vi "Izhikevich_primitive_v001.vi"(0 "UDP Network Connection in":refnum<k16>, 1 "b":dbl, 2 "a":dbl, 3 "I":dbl, 5 "c":dbl, 7 "d":dbl, 9 "v(t)":dbl, 10 "Neuron ID":dbl=1.0, 11 "error in (no error)":errorcluster, 12 "u(t)":dbl, 13 "dt":dbl) -> (4 "UDP Network Connection out":refnum<k16>, 6 "v(t+dt)":dbl, 8 "u(t+dt)":dbl, 15 "error out":errorcluster)   [LabVIEW 2019]
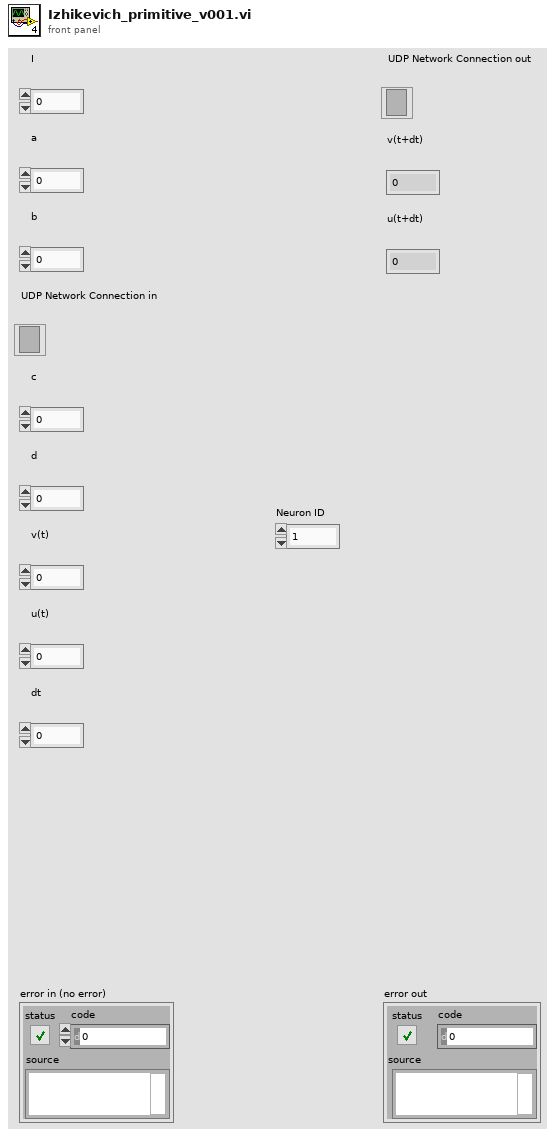
[diagram p1: front panel]
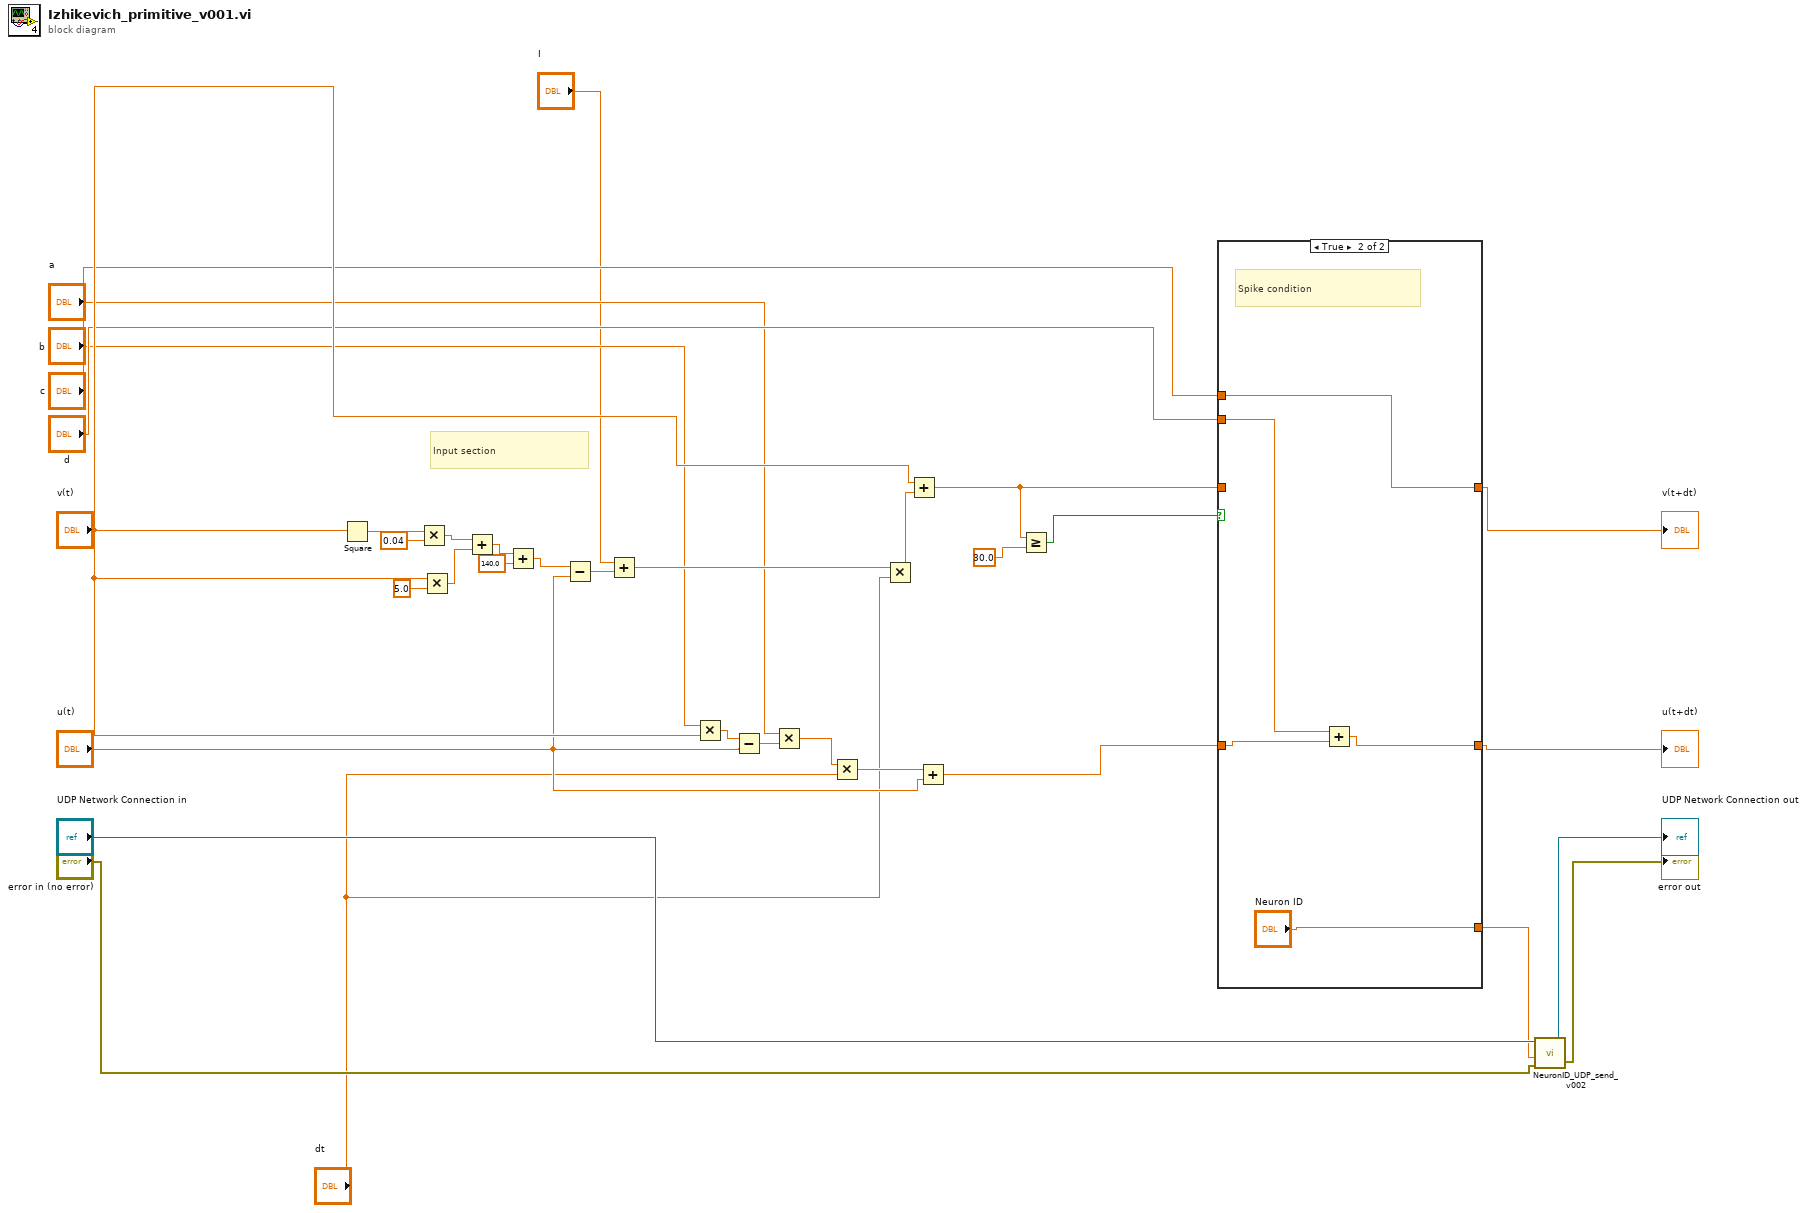
[diagram p0: block diagram]
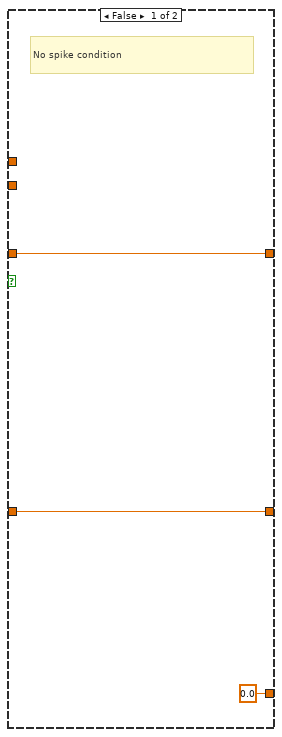
[diagram p2: hidden frame]
diagram:
  # "Input section"
  n1 = Square(x="v(t)") -> (x^2=w4:dbl)
  n2 = Multiply(x=w4, y=0.04) -> (x*y=w6:dbl)
  n3 = Multiply(x="v(t)", y=5.0) -> (x*y=w8:dbl)
  n4 = Add(x=w6, y=w8) -> (x+y=w9:dbl)
  n5 = Add(x=w9, y=140.0) -> (x+y=w11:dbl)
  n6 = Subtract(x=w11, y="u(t)") -> (x-y=w12:dbl)
  n7 = Add(x="I", y=w12) -> (x+y=w19:dbl)
  n8 = Multiply(x="b", y="v(t)") -> (x*y=w15:dbl)
  n9 = Subtract(x=w15, y="u(t)") -> (x-y=w16:dbl)
  n10 = Multiply(x="a", y=w16) -> (x*y=w18:dbl)
  n11 = Multiply(x=w18, y="dt") -> (x*y=w22:dbl)
  n12 = Multiply(x=w19, y="dt") -> (x*y=w21:dbl)
  n13 = Add(x="v(t)", y=w21) -> (x+y=w31:dbl)
  n14 = Add(x=w22, y="u(t)") -> (x+y=w24:dbl)
  n15 = Greater Or Equal?(x=w31, y=30.0) -> (x >= y?=w32:bool)
  n16 = case shown="True" w32 {
    tunnel: [w37 w39] -> w23
    tunnel: w24 -> [w37 w41]
    tunnel: w31 -> [w36 _]
    tunnel: [w36 w42] -> w25
    tunnel: "c" -> [_ w42]
    tunnel: "d" -> [_ w40]
    tunnel: [0.0 ("Neuron ID") "Neuron ID"] -> w3
    frame False {
      # "No spike condition"
    }
    frame True {
      # "Spike condition"
      n17 = Add(x=w40, y=w41) -> (x+y=w39:dbl)
    }
  }
  "v(t+dt)" <- w25
  "u(t+dt)" <- w23
  n18 = call "NeuronID_UDP_send_v002.vi"("error in (no error)"="error in (no error)", "Time"=w3, "UDP Network Connection in"="UDP Network Connection in") -> ("error out"=→"error out":errorcluster, "UDP Network Connection out"=→"UDP Network Connection out":refnum<k16>)  [unwired: 1 in]
